vi "Error Cluster from Error Code.vi"(5 "is warning? (False)":bool, 7 "show call chain? (False)":bool, 8 "Error In":errorcluster, 10 "Error Message (\"\")":string, 11 "Error Code (0)":i32) -> (0 "Error Out":errorcluster)   [LabVIEW 2015, in "CS++Utilities.lvlib"]
doc: "Converts an error or warning code to an error cluster.\n\n<B>Error Message</B> is the error description to appear in the <B>error out</B> cluster. It becomes appended to the error source string."
uses:
  CS++Utilities.lvlib
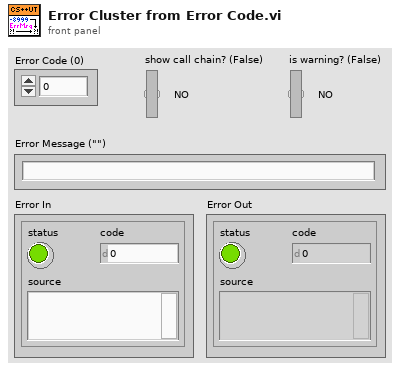
[diagram p1: front panel]
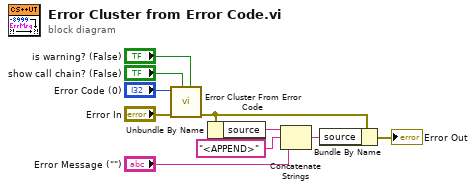
[diagram p0: block diagram]
diagram:
  n1 = call <vilib>:"Error Cluster From Error Code.vi"("is warning? (False)"="is warning? (False)", "show call chain? (False)"="show call chain? (False)", "error in (no error)"="Error In", "error code (0)"="Error Code (0)") -> ("error out"=w3:errorcluster)  [unwired: 5 in]
  n2 = Unbundle By Name(w3) -> ("source"=w10:string)
  n3 = Concatenate Strings(w10, "<APPEND>" ("string"), "Error Message (\"\")") -> (w9:string)
  n4 = Bundle By Name(cluster=w3, "source"=w9) -> (→"Error Out":errorcluster)
